vi "曲线拟合作业.vi"() -> ()   [LabVIEW 2014]
uses:
  <vilib>/Analysis/NI_AALBase.lvlib
  <vilib>/Analysis/NI_AALPro.lvlib
panel:
  out "数组":dbl[](array[numeric])
  out "XY图":cluster{dbl[], "Best Fit":dbl[]}[](graph)
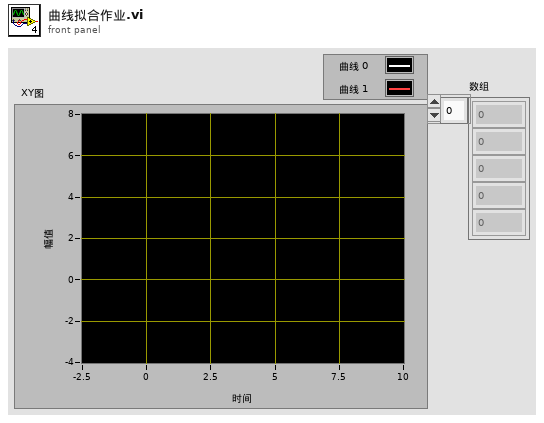
[diagram p1: front panel]
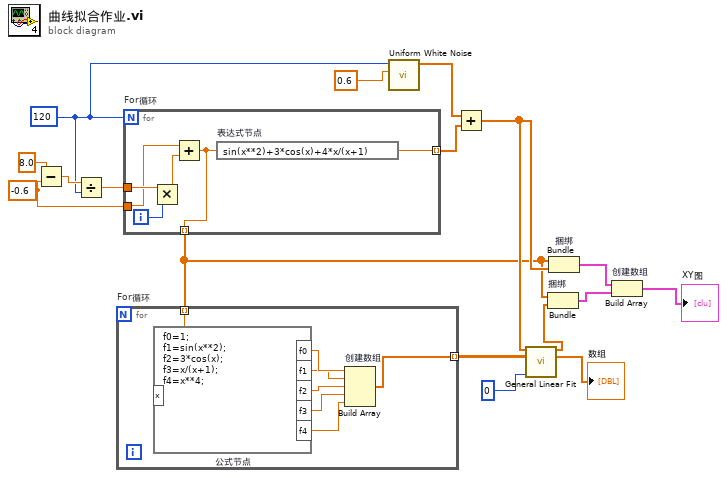
[diagram p0: block diagram]
diagram:
  w11 = 120
  w14 = -0.6
  n1 = Subtract(x=8.0, y=w14) -> (x-y=w16:dbl)
  n2 = Divide(x=w16, y=w11) -> (x/y=w15:dbl)
  n3 = for "For循环" {
    N: w11 -> [_]
    tunnel: w15 -> [w22]
    tunnel: w14 -> [w21]
    tunnel: [w20] -> w13 mode=indexing
    tunnel: [w18] -> w6 mode=indexing
    i -> [w23]
    n4 = Multiply(x=w22, y=w23) -> (x*y=w19:dbl)
    n5 = Add(x=w21, y=w19) -> (x+y=w18:dbl)
    n6 = expression code="sin(x**2)+3*cos(x)+4*x/(x+1)" "表达式节点"(w18) -> (w20:dbl)
  }
  n7 = for "For循环" {
    tunnel: w6 -> [w30] mode=indexing
    tunnel: [w24] -> w5 mode=indexing
    n8 = formula code="f0=1;\nf1=sin(x**2);\nf2=3*cos(x);\nf3=x/(x+1);\nf4=x**4;" "公式节点"("x"=w30) -> ("f0"=w29:dbl, "f1"=w28:dbl, "f2"=w27:dbl, "f3"=w26:dbl, "f4"=w25:dbl)
    n9 = Build Array "创建数组"(w29, w28, w27, w26, w25) -> (w24:dbl[])
  }
  n10 = call <vilib>:"Uniform White Noise.vi"("amplitude"=0.6, "samples"=w11) -> ("uniform white noise"=w10:dbl[])  [unwired: 8 in, 1 out]
  n11 = Add(x=w10, y=w13) -> (x+y=w8:dbl[])
  n12 = call <vilib>:"General Linear Fit.vi"("Y"=w8, "H"=w5, "method"=0) -> ("Best Fit"=w7:dbl[], "Coefficients"=→"数组":dbl[])  [unwired: 7 in, 4 out]
  n13 = Bundle "捆绑"(w6, "Best Fit"=w7) -> (w3:cluster{dbl[], "Best Fit":dbl[]})  [unwired: 1 in]
  n14 = Bundle "捆绑"(w6, w8) -> (w4:cluster{dbl[], dbl[]})  [unwired: 1 in]
  n15 = Build Array "创建数组"(w4, w3) -> (→"XY图":cluster{dbl[], "Best Fit":dbl[]}[])
